vi "MQTT-HomeAssistant-Discovery.vi"(0 "TCP Network Connection in":refnum<k5>, 1 "Device":string="cRIO_1", 2 "DeviceName":string="SaunaTemp", 3 "ChannelBase":string="Temp", 4 "ChannelNames":string[](array[string])=["SaunaHeaterTemp", "SaunaRoofTemp", "SaunaBenchTemp", "SaunaFloorTemp"], 5 "error in (no error)":errorcluster, 6 "Publish Meta":cluster{"QoS":T1, "Retain":T2, "DUP":T3}) -> (14 "TCP Network Connection out":refnum<k5>, 15 "Topics":string[](array[string]), 19 "error out":errorcluster)   [LabVIEW 2024]
uses:
  LVMQTT-master/Controls/QoS.ctl
  LVMQTT-master/Controls/Retain_Flag.ctl
  LVMQTT-master/Controls/DUP_Flag.ctl
  LVMQTT-master/MQTT_Functions.lvlib
panel:
  out "Array":errorcluster[](array[cluster])
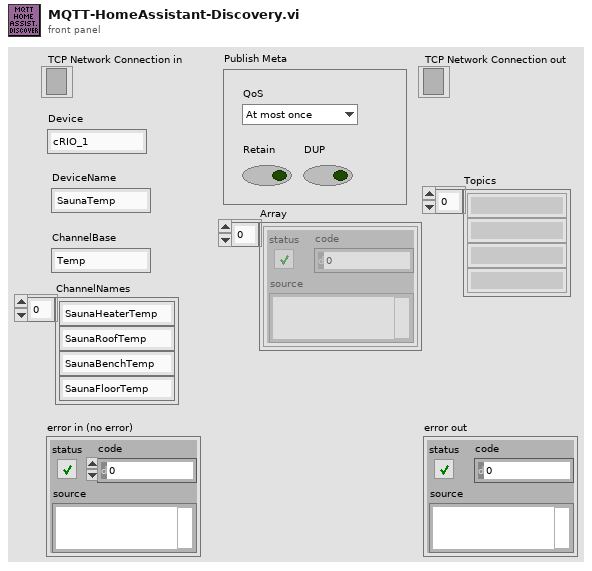
[diagram p1: front panel]
types:
  T1 = typedef "MQTT_Functions.lvlib/QoS.ctl" = enum8{"At most once", "At least once", "Exactly once", "Reserved"}
  T2 = typedef "MQTT_Functions.lvlib/Retain_Flag.ctl" = bool
  T3 = typedef "MQTT_Functions.lvlib/DUP_Flag.ctl" = bool
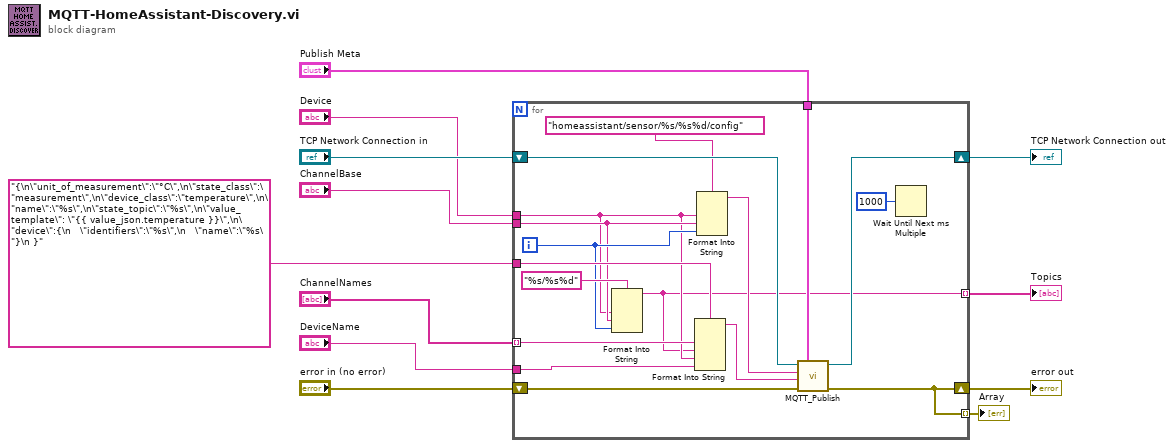
[diagram p0: block diagram]
diagram:
  n1 = for {
    shift-right: [w13] -> w12
    shift-left: "error in (no error)" -> [w29]
    shift-right: [w28] -> w10
    shift-left: "TCP Network Connection in" -> [w27]
    tunnel: "Publish Meta" -> [w26]
    tunnel: "Device" -> [w18]
    tunnel: "ChannelBase" -> [w19]
    tunnel: "{\n\"unit_of_measurement\":\"°C\",\n\"state_class\":\"measurement\",\n\"device_class\":\"temperature\",\n\"name\":\"%s\",\n\"state_topic\":\"%s\",\n\"value_template\": \"{{ value_json.temperature }}\",\n\"device\":{\n   \"identifiers\":\"%s\",\n   \"name\":\"%s\"}\n }" -> [w23]
    tunnel: "ChannelNames" -> [w22] mode=indexing
    tunnel: "DeviceName" -> [w17]
    tunnel: [w16] -> w2 mode=indexing
    tunnel: [w13] -> w1 mode=indexing
    i -> [w20]
    n2 = Format Into String(format string="%s/%s%d", w18, w19, w20) -> (resulting string=w16:string)  [unwired: 2 in, 1 out]
    n3 = Format Into String(format string=w23, w22, w16, w18, w17) -> (resulting string=w15:string)  [unwired: 2 in, 1 out]
    n4 = Format Into String(format string="homeassistant/sensor/%s/%s%d/config", w18, w19, w20) -> (resulting string=w24:string)  [unwired: 2 in, 1 out]
    n5 = call "MQTT_Publish.vi"("Publish Meta"=w26, "error in (no error)"=w29, "Message to be published"=w15, "Topic"=w24, "connection ID"=w27) -> ("error out"=w13:errorcluster, "connection ID out"=w28:refnum<k5>)  [unwired: 5 in]
    n6 = Wait Until Next ms Multiple(millisecond multiple=u32 1000) -> ()  [unwired: 1 out]
  }
  "error out" <- w12
  "TCP Network Connection out" <- w10
  "Topics" <- w2
  "Array" <- w1
